vi "Zigbee_CRC16_Calculator.vi"(5 "ByteOrder":bool=TRUE, 6 "ReverseCRC":bool=TRUE, 7 "LSB First":bool=TRUE, 8 "Postcond":bool=TRUE, 9 "Precond":bool=TRUE, 10 "Polynom":u16=4129 format="%.0x", 11 "Input":u8[](array[numeric]) format="%x") -> (1 "Bytes":u8[](array[numeric]) format="%.0x", 2 "Numeric":u16 format="%.0x", 3 "CRC16 out":string)   [LabVIEW 2020]
doc: "This is a general 16 bit CRC calculation VI.\n\nThe standard inputs will calculate the CRC with the following conditions:\n\nPolynom: x^16+x^12+x^5+1\nPrecondition: 0x0000\nPostcondition: not inverting\nMost significant bit of a byte first\nCRC output not bitwise reversed\nMost significant byte first\n\nThe input \"Check this message!\" will generate an output of 0x9E8F.\n\nThe VI was started by Shane aka shoneill in the NI Developer Zone. He implemented the HW like algorithm in the inner loop. Many thanks to him.\n\nThis VI was created and tested for the Intel plattform. I'm not sure that the byte order will be correct on a Motorola plattform."
panel:
  # "Input"
  # "Output"
  # "Conditioning"
  # "Bitsequence"
  # "Output Byte Order"
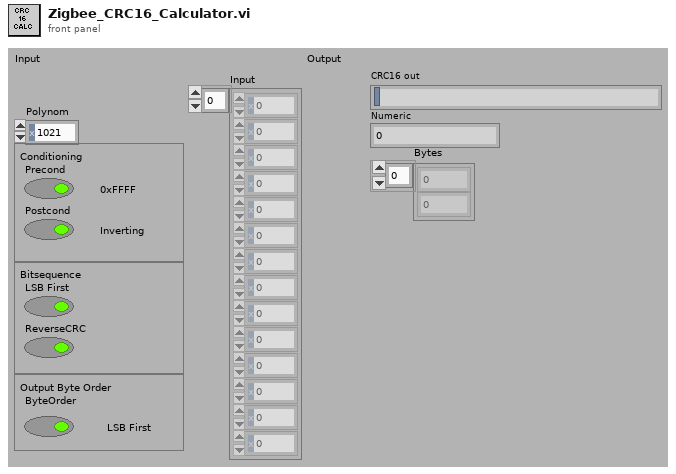
[diagram p1: front panel]
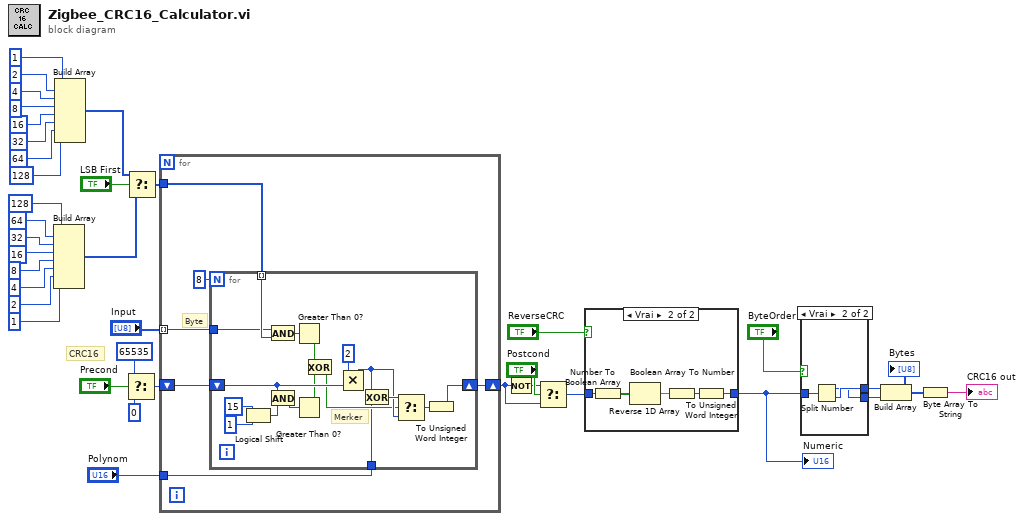
[diagram p0: block diagram]
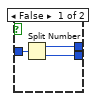
[diagram p2: hidden frame]
diagram:
  # "CRC16"
  n1 = Build Array(u8 128, u8 64, u8 32, u8 16, u8 8, u8 4, u8 2, u8 1) -> (w16:u8[])
  n2 = Build Array(u8 1, u8 2, u8 4, u8 8, u8 16, u8 32, u8 64, u8 128) -> (w15:u8[])
  n3 = Select(t=u16 65535, s="Precond", f=u16 0) -> (s? t:f=w37:u16)
  n4 = Select(t=w15, s="LSB First", f=w16) -> (s? t:f=w18:u8[])
  n5 = for {
    shift-right: [w41] -> w12
    shift-left: w37 -> [w43]
    tunnel: "Input" -> [w40] mode=indexing
    tunnel: w18 -> [w39]
    tunnel: "Polynom" -> [w38]
    # "Byte"
    n6 = for {
      N: 8 -> [_]
      shift-right: [w59] -> w41
      shift-left: w43 -> [w49]
      tunnel: w39 -> [w50] mode=indexing
      tunnel: w40 -> [w45]
      tunnel: w38 -> [w44]
      # "Merker"
      n7 = Logical Shift(y=u16 15, x=u16 1) -> (x << y=w53:u16)
      n8 = And(x=w45, y=w50) -> (x .and. y?=w57:u8)
      n9 = And(x=w49, y=w53) -> (x .and. y?=w52:u16)
      n10 = Greater Than 0?(x=w57) -> (x > 0?=w56:bool)
      n11 = Greater Than 0?(x=w52) -> (x > 0?=w47:bool)
      n12 = Exclusive Or(1:w47, 2:w56) -> (0:w46:bool)
      n13 = Multiply(x=u16 2, y=w49) -> (x*y=w51:u16)
      n14 = Exclusive Or(1:w44, 2:w51) -> (0:w60:u16)
      n15 = Select(t=w60, s=w46, f=w51) -> (s? t:f=w58:u16)
      n16 = To Unsigned Word Integer(number=w58) -> (unsigned 16bit integer=w59:u16)
    }
  }
  n17 = Not(x=w12) -> (.not. x?=w11:u16)
  n18 = Select(t=w11, s="Postcond", f=w12) -> (s? t:f=w10:u16)
  n19 = case shown="Vrai" "ReverseCRC" {
    tunnel: w10 -> [w61 w66]
    tunnel: [w61 w62] -> w2
    frame False {
    }
    frame True {
      n20 = Number To Boolean Array(number=w66) -> (Boolean array=w65:bool[])
      n21 = Reverse 1D Array(array=w65) -> (reversed array=w64:bool[])
      n22 = Boolean Array To Number(Boolean array=w64) -> (number=w63:u32)
      n23 = To Unsigned Word Integer(number=w63) -> (unsigned 16bit integer=w62:u16)
    }
  }
  "Numeric" <- w2
  n24 = case shown="Vrai" "ByteOrder" {
    tunnel: w2 -> [w69 w72]
    tunnel: [w68 w71] -> w3
    tunnel: [w67 w70] -> w4
    frame False {
      n25 = Split Number(x=w69) -> (hi(x)=w68:u8, lo(x)=w67:u8)
    }
    frame True {
      n26 = Split Number(x=w72) -> (hi(x)=w70:u8, lo(x)=w71:u8)
    }
  }
  n27 = Build Array(w3, w4) -> (w6:u8[])
  "Bytes" <- w6
  n28 = Byte Array To String(unsigned byte array=w6) -> (string=→"CRC16 out":string)
